vi "GetWindowProperties.vi"(8 "No Error":errorcluster, 11 "Window [SDL_Window *]":i64 format="%.0x") -> (0 "Error Out":errorcluster, 3 "PropertiesID":T1)   [LabVIEW 2024, in "SDL3.lvlib" / "Video.lvlib"]
doc: "<B>Summary</B>\nGet the properties associated with a window.\n\n<B>Remarks</B>\nThe following read-only properties are provided by SDL:\n\n- <B>SDL_PROP_WINDOW_SHAPE_POINTER</B>: the surface associated with a shaped window\n- <B>SDL_PROP_WINDOW_HDR_ENABLED_BOOLEAN</B>: true if the window has HDR headroom above the SDR white point. This property can change dynamically when - <B>SDL_EVENT_WINDOW_HDR_STATE_CHANGED</B> is sent.\n- <B>SDL_PROP_WINDOW_SDR_WHITE_LEVEL_FLOAT</B>: the value of SDR white in the - <B>SDL_COLORSPACE_SRGB_LINEAR</B> colorspace. On Windows this corresponds to the SDR white level in scRGB colorspace, and on Apple platforms this is always 1.0 for EDR content. This property can change dynamically when <B>SDL_EVENT_WINDOW_HDR_STATE_CHANGED</B> is sent.\n- <B>SDL_PROP_WINDOW_HDR_HEADROOM_FLOAT</B>: the additional high dynamic range that can be displayed, in terms of the SDR white point. When HDR is not enabled, this will be 1.0. This property can change dynamically when <B>SDL_EVENT_WINDOW_HDR_STATE_CHANGED</B> is sent.\n\nOn Windows:\n- <B>SDL_PROP_WINDOW_WIN32_HWND_POINTER</B>: the HWND associated with the window\n- <B>SDL_PROP_WINDOW_WIN32_HDC_POINTER</B>: the HDC associated with the window\n- <B>SDL_PROP_WINDOW_WIN32_INSTANCE_POINTER</B>: the HINSTANCE associated with the window\n\nOn Wayland:\nNote: The xdg_* window objects do not internally persist across window show/hide calls. They will be null if the window is hidden and must be queried each time it is shown.\n\n- <B>SDL_PROP_WINDOW_WAYLAND_DISPLAY_POINTER</B>: the wl_display associated with the window\n- <B>SDL_PROP_WINDOW_WAYLAND_SURFACE_POINTER</B>: the wl_surface associated with the window\n- <B>SDL_PROP_WINDOW_WAYLAND_VIEWPORT_POINTER</B>: the wp_viewport associated with the window\n- <B>SDL_PROP_WINDOW_WAYLAND_EGL_WINDOW_POINTER</B>: the wl_egl_window associated with the window\n- <B>SDL_PROP_WINDOW_WAYLAND_XDG_SURFACE_POINTER</B>: the xdg_surface associated with the window\n- <B>SDL_PROP_WINDOW_WAYLAND_XDG_TOPLEVEL_POINTER</B>: the xdg_toplevel role associated with the window\n- <B>SDL_PROP_WINDOW_WAYLAND_XDG_TOPLEVEL_EXPORT_HANDLE_STRING</B>: the export handle associated with the window\n- <B>SDL_PROP_WINDOW_WAYLAND_XDG_POPUP_POINTER</B>: the xdg_popup role associated with the window\n- <B>SDL_PROP_WINDOW_WAYLAND_XDG_POSITIONER_POINTER</B>: the xdg_positioner associated with the window, in popup mode\n\nOn X11:\n- <B>SDL_PROP_WINDOW_X11_DISPLAY_POINTER</B>: the X11 Display associated with the window\n- <B>SDL_PROP_WINDOW_X11_SCREEN_NUMBER</B>: the screen number associated with the window\n- <B>SDL_PROP_WINDOW_X11_WINDOW_NUMBER</B>: the X11 Window associated with the window"
uses:
  Video.lvlib
  Properties/PropertiesID--integer.ctl
  <vilib>/Utility/error.llb/Error Cluster From Error Code.vi
  Lib/SDL3-32.dll
  Error/Error.lvlib
  Properties/Properties.lvlib
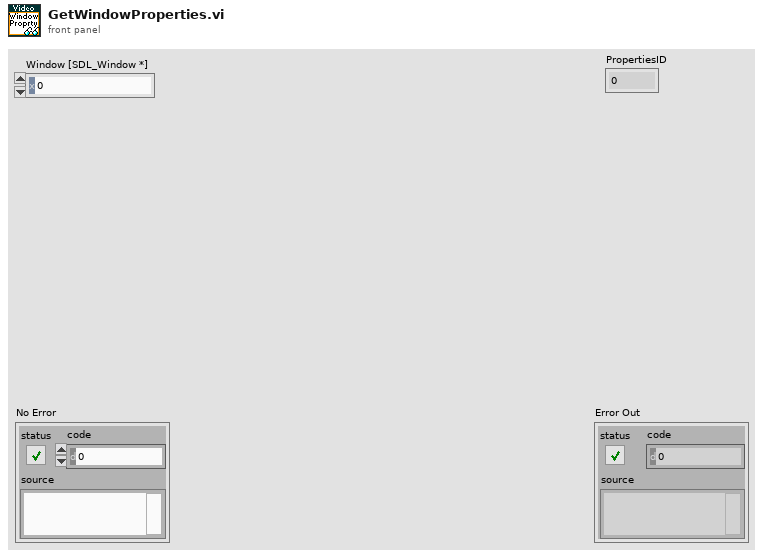
[diagram p1: front panel]
types:
  T1 = typedef "SDL3.lvlib/Properties.lvlib/PropertiesID--integer.ctl" = u32
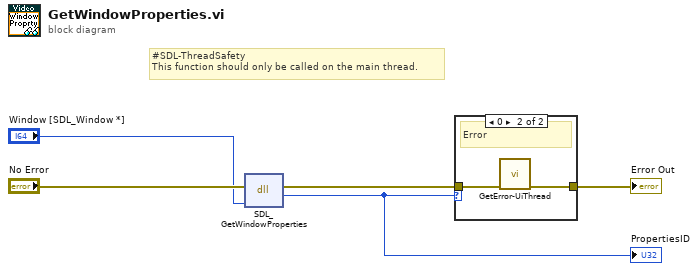
[diagram p0: block diagram]
diagram:
  # "#SDL-ThreadSafety\nThis function should only be called on the main thread."
  n1 = dll-call lib="C:/Users/Thomas/Documents/Projects/LV-SDL3/Lib/SDL3-*.*" fn="SDL_GetWindowProperties"(error in="No Error", "window"="Window [SDL_Window *]") -> (error out=w2:errorcluster, "return type"=w1:u32)  [unwired: 3 in, 1 out]
  "PropertiesID" <- w1
  n2 = case shown="0" w1 {
    tunnel: w2 -> [w6 w8]
    tunnel: [w6 w7] -> w4
    frame Default {
      # "Ok"
    }
    frame 0 {
      # "Error"
      n3 = call "GetError-UiThread.vi"("No Error"=w8) -> ("error out"=w7:errorcluster)  [unwired: 10 in]
    }
  }
  "Error Out" <- w4
